vi "sio lctrl.vi"(8 "mode":i32, 11 "port":i32) -> (0 "Status":i32, 3 "port":i32)   [LabVIEW 2015, in "PCOMM.lvlib"]
doc: "int WINAPI sio_close(int port);\nMode: DTR_state OR RTS_state. 0= Off, 1=On. (0x00, 0x01, 0x02, 0x03)\n bit0 STR state/ bit1 RTS states"
uses:
  PCOMM.lvlib
  PCOMM.DLL
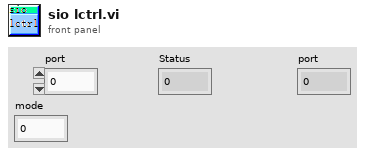
[diagram p1: front panel]
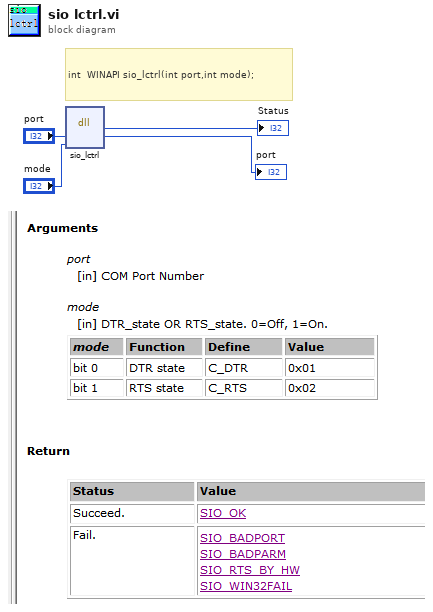
[diagram p0: block diagram]
diagram:
  # "int  WINAPI sio_lctrl(int port,int mode);"
  n1 = dll-call lib="PTH2^abs EDesktopLabview串口助手串口助手2.0Ing10_v3.2.0SubVIpcomm库PCOMM.*" fn="sio_lctrl"("port"="port", "mode"="mode") -> ("返回类型"=→"Status":i32, "port"=→"port":i32)  [unwired: 4 in, 2 out]
